vi "Service map delete.vi"(4 "error in (no error)":errorcluster, 6 "Index":i32, 7 "CANopen in":refnum<class "CANopen.lvclass">) -> (0 "error out":errorcluster, 3 "CANopen out":refnum<class "CANopen.lvclass">)   [LabVIEW 2026, in "canopen_.lvlib" / "CANopen.lvclass"]
doc: "Deletes a specific entry from the service map. The deletion is protected with a mutex in order to prevent race conditions with \"Service map insert\"."
uses:
  CANopen.lvclass
  CANopen.lvclass/CANopen.ctl
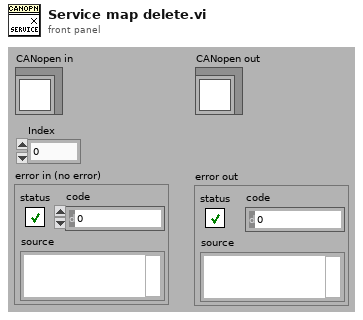
[diagram p1: front panel]
types:
  T1 = typedef "Semaphore RefNum" = refnum<k1>
  T2 = cluster{"CobID":u32, "Data offset":u8, "Data size":u8, "Destination":refnum<vi>}[]
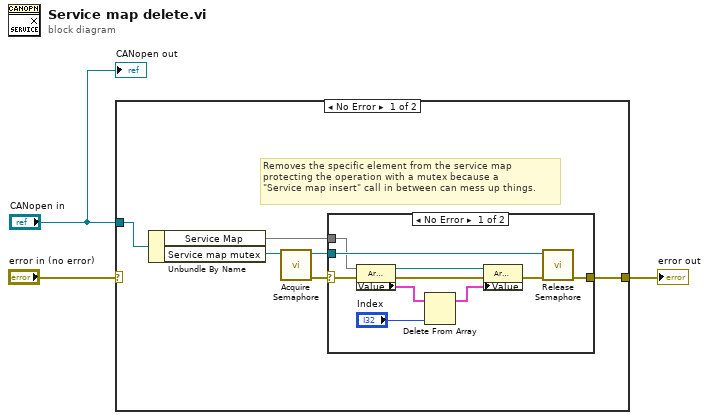
[diagram p0: block diagram]
diagram:
  n1 = case shown="No Error" "error in (no error)" {
    selector: "error in (no error)" -> [_ w21]
    tunnel: [w9 w21] -> w3
    tunnel: "CANopen in" -> [w7 _]
    frame No Error {
      # "Removes the specific element from the service map\nprotecting the operation with a mutex because a\n\"Service map insert\" call in between can mess up things."
      n2 = Unbundle By Name(w7) -> ("Service Map"=w5:map{u32, u8[]}, "Service map mutex"=w6:T1)
      n3 = call <vilib>:"Acquire Semaphore.vi"("semaphore"=w6) -> ("error out"=w4:errorcluster, "semaphore out"=w8:T1)  [unwired: 2 in, 3 out]
      n4 = case shown="No Error" w4 {
        selector: w4 -> [w10 w20]
        tunnel: [w16 w20] -> w9
        tunnel: w8 -> [w13 _]
        tunnel: w5 -> [w12 _]
        frame No Error {
          n5 = property class="Arr (strict)"(reference=w12, error in=w10) -> (reference out=w11:refnum<vi>, error out=w14:errorcluster, "Value"=w15:T2)
          n6 = Delete From Array(array=w15, index="Index") -> (array with subset deleted=w19:T2)  [unwired: 1 in, 1 out]
          n7 = property class="Arr (strict)"(reference=w11, error in=w14, "Value"=w19) -> (error out=w17:errorcluster)  [unwired: 1 out]
          n8 = call <vilib>:"Release Semaphore.vi"("error in (no error)"=w17, "semaphore"=w13) -> ("error out"=w16:errorcluster)  [unwired: 5 out]
        }
        frame Error {
        }
      }
    }
    frame Error {
    }
  }
  "error out" <- w3
  "CANopen out" <- "CANopen in"
